vi "Refresh DQMH Module By Name.vi"(8 "error in":errorcluster, 9 "Event Type (New)":T1, 10 "Event Name":string, 11 "DQMH Lib Name":string) -> (0 "error out":errorcluster)   [LabVIEW 2019, in "Panther Dashboard.lvlib"]
doc: "Refresh DMQH Module by name, this is going to be used with the NEW <b> Scripting Hooks DQMH 7.1 Feature </b>\n\n_____\nCreated using DQMH Event Scripter 7.1.0.1447."
uses:
  Panther Dashboard.lvlib
  Refresh DQMH Module By Name Argument--cluster.ctl
  <vilib>/Delacor/Delacor QMH/Libraries/_Scripting Support/Event Type (New)--enum.ctl
  <vilib>/Delacor/Delacor QMH/Libraries/_Scripting Support/dqmh_lib_DQMH Scripting Support.lvlib
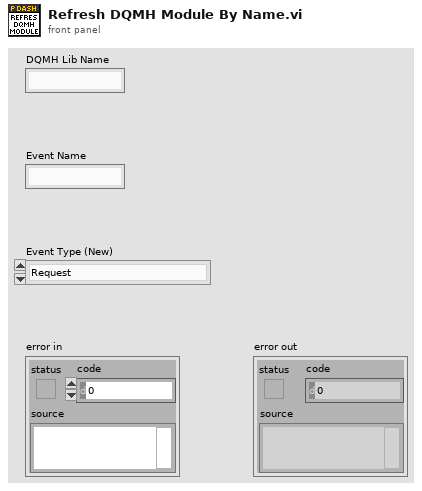
[diagram p1: front panel]
types:
  T1 = typedef "dqmh_lib_DQMH Scripting Support.lvlib/Event Type (New)--enum.ctl" = enum16{"Request", "Broadcast", "Request and Wait for Reply", "Round Trip"}
  T2 = typedef "Panther Dashboard.lvlib/Refresh DQMH Module By Name Argument--cluster.ctl" = cluster{"Event Type (New)":T1, "DQMH Lib Name":string, "Event Name":string}
  T3 = typedef "Panther Dashboard.lvlib/Request Events--cluster.ctl" = cluster{"Stop Module":refnum<user-event>, "Show Panel":refnum<user-event>, "Hide Panel":refnum<user-event>, "Get Module Execution Status":refnum<user-event>, "Show Diagram":refnum<user-event>, "Scan DQMH Modules":refnum<user-event>, "Tree DQMH Selection":refnum<user-event>, "Open Module API Tester":refnum<user-event>, "Execute Default Event Request":refnum<user-event>, "Launch DQMH Scripting Tools":refnum<user-event>, "Generate Project Documentation":refnum<user-event>, "Show About":refnum<user-event>, "Update Module ID":refnum<user-event>, "Save Library Description":refnum<user-event>, "Save VI Description":refnum<user-event>, "Open Documentation":refnum<user-event>, "Save Project Documentation":refnum<user-event>, "Register controls Mouse Enter":refnum<user-event>, "Load Project From Path":refnum<user-event>, "Add DQMH Module to Current Scan":refnum<user-event>, "Refresh DQMH Module By Name":refnum<user-event>}
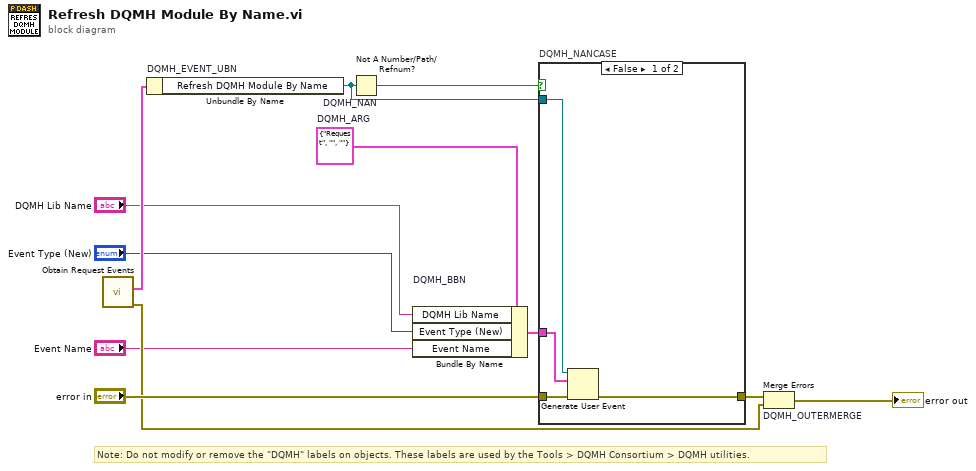
[diagram p0: block diagram]
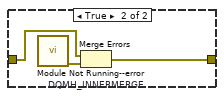
[diagram p2: hidden frame]
diagram:
  w5 = T2 {"Event Type (New)"=enum."Request", "DQMH Lib Name"="", "Event Name"=""}  # DQMH_ARG
  # "Note: Do not modify or remove the \"DQMH\" labels on objects. These labels are used by the Tools > DQMH Consortium > DQMH utilities."
  n1 = call "Obtain Request Events.vi"() -> ("error out"=w9:errorcluster, "Panther Dashboard Request Events"=w4:T3)  [unwired: 10 in]
  n2 = Unbundle By Name "DQMH_EVENT_UBN"(w4) -> ("Refresh DQMH Module By Name"=w6:refnum<user-event>)
  n3 = Not A Number/Path/Refnum? "DQMH_NAN"(number/path/refnum=w6) -> (NaN/Path/Refnum?=w7:bool)
  n4 = Bundle By Name "DQMH_BBN"(cluster=w5, "DQMH Lib Name"="DQMH Lib Name", "Event Type (New)"="Event Type (New)", "Event Name"="Event Name") -> (w8:T2)
  n5 = case "DQMH_NANCASE" shown="False" w7 {
    tunnel: "error in" -> [w16 w19]
    tunnel: [w15 w18] -> w10
    tunnel: w6 -> [w14 _]
    tunnel: w8 -> [w13 _]
    frame False {
      n6 = Generate User Event(user event=w14, event data cluster=w13, error in=w16) -> (error out=w15:errorcluster)  [unwired: 1 in, 1 out]
    }
    frame True {
      n7 = call "Module Not Running--error.vi"() -> ("error out"=w17:errorcluster)  [unwired: 11 in]
      n8 = Merge Errors "DQMH_INNERMERGE"(w19, w17) -> (w18:errorcluster)
    }
  }
  n9 = Merge Errors "DQMH_OUTERMERGE"(w10, w9) -> (→"error out":errorcluster)
